vi "Set Title.vi"(8 "error in (no error)":errorcluster, 10 "Title":string="Simon's UI Demo", 11 "DemoMain in":refnum<class "DemoMain.lvclass">) -> (0 "error out":errorcluster, 3 "DemoMain out":refnum<class "DemoMain.lvclass">)   [LabVIEW 2012, in "Win8uiDemo.lvlib" / "DemoMain.lvclass"]
uses:
  DemoMain.lvclass
  Win8uiFramework/MainController.lvclass
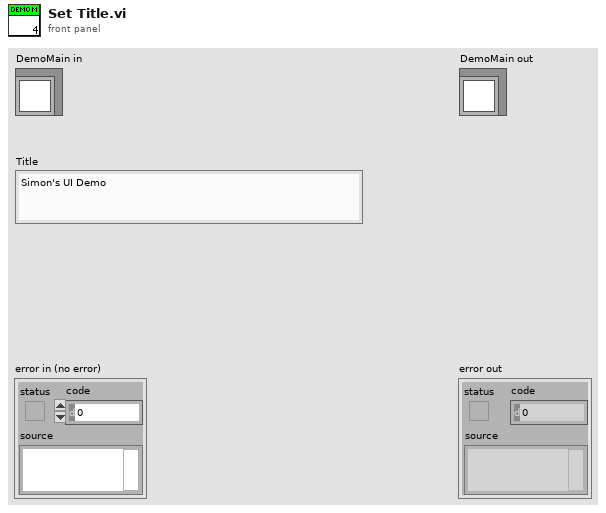
[diagram p1: front panel]
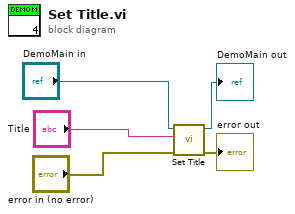
[diagram p0: block diagram]
diagram:
  n1 = call-parent "Set Title.vi"("error in (no error)"="error in (no error)", "Title"="Title", "MainController in"="DemoMain in") -> ("error out"=→"error out":errorcluster, "MainController out"=→"DemoMain out":refnum<class "DemoMain.lvclass">)  [unwired: 7 in]
